vi "Test Filter read.vi"   [LabVIEW 2012]
uses:
  <vilib>/DAQmx/write.llb/DAQmx Write (Digital 1D Bool NChan 1Samp 1Line).vi
  Reusable/Serial IO/Serial IO.lvclass
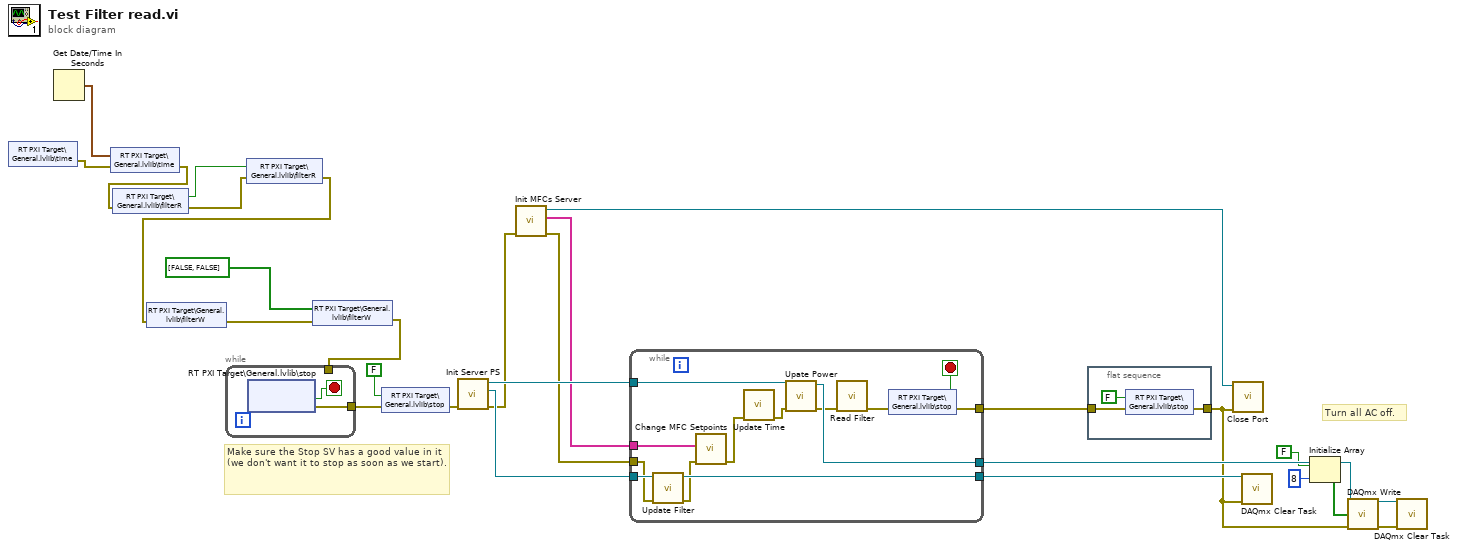
[diagram p0: block diagram]
diagram:
  # "Make sure the Stop SV has a good value in it (we don't want it to stop as soon as we start)."
  # "Turn all AC off."
  n1 = shared-variable "RT PXI Target\\General.lvlib\\time"() -> (error out=w5:errorcluster)  [unwired: 1 in, 1 out]
  n2 = Get Date/Time In Seconds() -> (seconds since 1Jan1904=w6:timestamp)
  n3 = shared-variable "RT PXI Target\\General.lvlib\\time"(w6, error in=w5) -> (error out=w4:errorcluster)
  n4 = shared-variable "RT PXI Target\\General.lvlib\\filterR"(error in=w4) -> (w2:bool, error out=w3:errorcluster)
  n5 = shared-variable "RT PXI Target\\General.lvlib\\filterR"(w2, error in=w3) -> (error out=w1:errorcluster)
  n6 = shared-variable "RT PXI Target\\General.lvlib\\filterW"(error in=w1) -> (error out=w8:errorcluster)  [unwired: 1 out]
  n7 = shared-variable "RT PXI Target\\General.lvlib\\filterW"(bool[] [FALSE, FALSE] ("filterW"), error in=w8) -> (error out=w7:errorcluster)
  n8 = while {
    tunnel: [w28] -> w24
    tunnel: w7 -> [_]
    stop <- w29 stop-if-true
    n9 = shared-variable "RT PXI Target\\General.lvlib\\stop"() -> (error out=w28:errorcluster, w29:bool)  [unwired: 2 in, 1 out]
  }
  n10 = shared-variable "RT PXI Target\\General.lvlib\\stop"(FALSE ("stop"), error in=w24) -> (error out=w23:errorcluster)
  n11 = call "Init Server PS.vi"("error in"=w23) -> ("error out"=w13:errorcluster, "Filter Out Task"=w16:refnum<k21>, "PS Switch Out"=w22:refnum<k21>)  [unwired: 8 in]
  n12 = call "Init MFCs Server.vi"("error in"=w13) -> ("error out"=w11:errorcluster, "Address Out"=w12:string[], "Serial IO out"=w10:refnum<class "Serial IO.lvclass">)  [unwired: 8 in]
  n13 = while {
    tunnel: [w41] -> w26
    tunnel: w22 -> [w40]
    tunnel: [w39] -> w25
    tunnel: w16 -> [w35]
    tunnel: [w34] -> w15
    tunnel: w11 -> [w32]
    tunnel: w12 -> [w37]
    stop <- w42 stop-if-true
    n14 = call "Update Filter.vi"("error in"=w32, "Refnum in"=w35) -> ("error out"=w33:errorcluster, "Refnum out"=w34:refnum<k21>)  [unwired: 8 in]
    n15 = call "Change MFC Setpoints.vi"("error in"=w33, "Address Out"=w37) -> ("error out"=w36:errorcluster)  [unwired: 8 in, 1 out]
    n16 = call "Update Time.vi"("error in"=w36) -> ("error out"=w38:errorcluster)  [unwired: 10 in]
    n17 = call "Upate Power.vi"("error in"=w38, "Refnum in"=w40) -> ("error out"=w31:errorcluster, "Refnum out"=w39:refnum<k21>)  [unwired: 8 in]
    n18 = call "Read Filter.vi"("error in"=w31) -> ("error out"=w30:errorcluster)  [unwired: 10 in]
    n19 = shared-variable "RT PXI Target\\General.lvlib\\stop"(error in=w30) -> (w42:bool, error out=w41:errorcluster)
  }
  n20 = flat-sequence {
    tunnel: w26 -> [w44]
    tunnel: [w43] -> w14
    frame #0 {
      n21 = shared-variable "RT PXI Target\\General.lvlib\\stop"(FALSE ("stop"), error in=w44) -> (error out=w43:errorcluster)
    }
  }
  n22 = call-dynamic "Close Port.vi"("error in (no error)"=w14, "Serial IO in"=w10) -> ()  [unwired: 8 in, 2 out]
  n23 = call <vilib>:"DAQmx Clear Task.vi"("task in"=w15, "error in"=w14) -> ()  [unwired: 13 in, 1 out]
  n24 = Initialize Array(FALSE, 8 ("dimension size")) -> (w19:bool[])
  n25 = call-poly <vilib>:"DAQmx Write.vi"("task/channels in"=w25, "data"=w19, "error in"=w14) -> ("task out"=w18:refnum<k21>, "error out"=w17:errorcluster)  [unwired: 10 in, 1 out]
  n26 = call <vilib>:"DAQmx Clear Task.vi"("task in"=w18, "error in"=w17) -> ()  [unwired: 13 in, 1 out]
